vi "c ctre phoenixpro serialize int no malloc.vi"(7 "max_len":u32, 8 "error in (no error)":errorcluster, 9 "str":string, 10 "value":i32, 11 "spn":i32) -> (0 "error out":errorcluster, 1 "str out":string, 3 "function return":i32)   [LabVIEW 2020, in "CTRE_PhoenixTools.lvlib"]
doc: "CTREXPORT int c_ctre_phoenixpro_serialize_int_no_malloc(int spn, int value, char *str, uint32_t max_len);"
uses:
  CTRE_PhoenixTools.lvlib
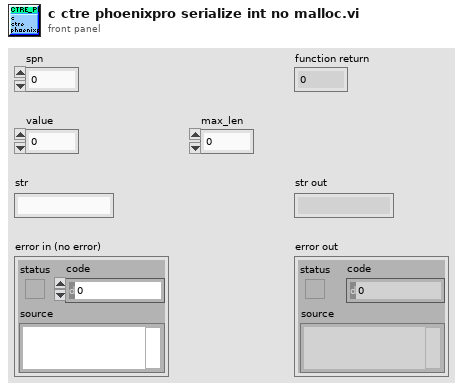
[diagram p1: front panel]
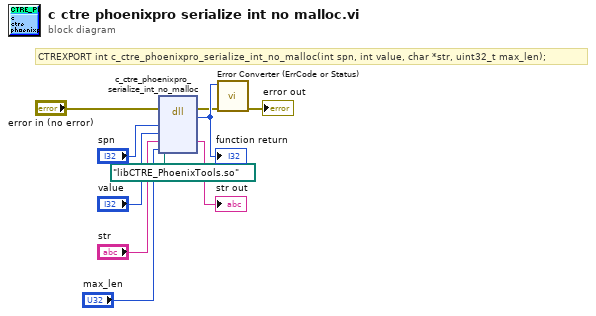
[diagram p0: block diagram]
diagram:
  # "CTREXPORT int c_ctre_phoenixpro_serialize_int_no_malloc(int spn, int value, char *str, uint32_t max_len);"
  n1 = dll-call lib="?" fn="c_ctre_phoenixpro_serialize_int_no_malloc"(path in=path "libCTRE_PhoenixTools.so", error in="error in (no error)", "spn"="spn", "value"="value", "str"="str", "max_len"="max_len") -> (error out=w3:errorcluster, w10:i32, "str"=→"str out":string)  [unwired: 4 in, 1 out]
  "function return" <- w10
  n2 = call "Error Converter (ErrCode or Status).vi"("error in (no error)"=w3, "error code"=w10) -> ("error out"=→"error out":errorcluster)  [unwired: 9 in]
